vi "CMD git branch -v.vi"(8 "error in (no error)":errorcluster, 10 "git repo path":path=path "C:/Users/user/Desktop", 11 "git.exe path":path=path "C:/Program Files/Git/cmd/git.exe") -> (0 "error out":errorcluster, 2 "standard error":string, 3 "standard output":string, 5 "command operated":string)   [LabVIEW 2016]
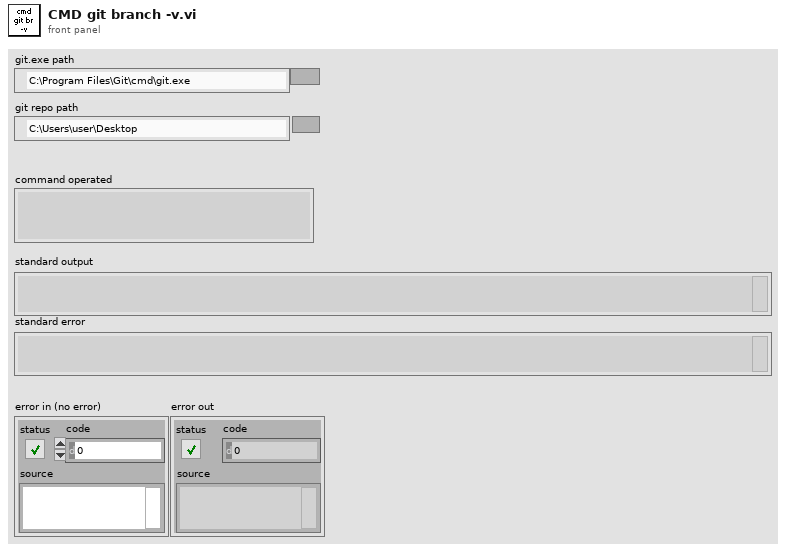
[diagram p1: front panel]
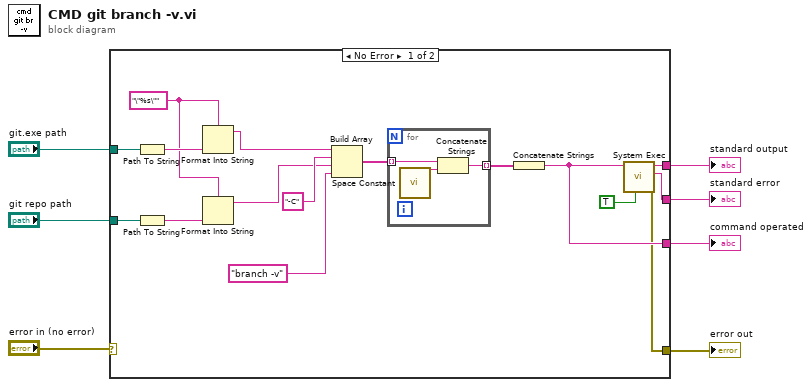
[diagram p0: block diagram]
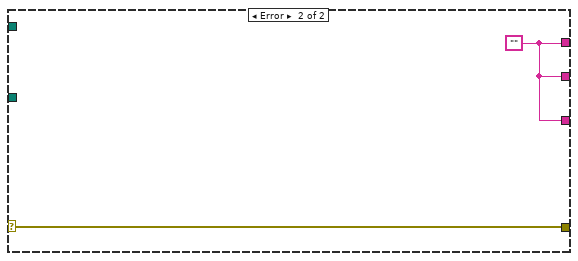
[diagram p2: hidden frame]
diagram:
  n1 = case shown="No Error" "error in (no error)" {
    selector: "error in (no error)" -> [_ w28]
    tunnel: "git repo path" -> [w19 _]
    tunnel: [w13 w27] -> w6
    tunnel: [w12 w27] -> w5
    tunnel: "git.exe path" -> [w10 _]
    tunnel: [w9 w27] -> w3
    tunnel: [w8 w28] -> w1
    frame No Error {
      w17 = "\"%s\"" ("format string")
      n2 = Path To String(path=w10) -> (string=w18:string)
      n3 = Path To String(path=w19) -> (string=w16:string)
      n4 = Format Into String(format string=w17, w18) -> (resulting string=w15:string)  [unwired: 2 in, 1 out]
      n5 = Format Into String(format string=w17, w16) -> (resulting string=w14:string)  [unwired: 2 in, 1 out]
      n6 = Build Array(w15, "-C" ("string"), w14, "branch -v" ("string")) -> (w21:string[])
      n7 = for {
        tunnel: w21 -> [w26] mode=indexing
        tunnel: [w24] -> w20 mode=indexing
        n8 = call <vilib>:"Space Constant.vi"() -> ("String"=w25:string)
        n9 = Concatenate Strings(w26, w25) -> (w24:string)
      }
      n10 = Concatenate Strings(w20) -> (w13:string)
      n11 = call <vilib>:"System Exec.vi"("run minimized? (F)"=TRUE, "command line"=w13) -> ("error out"=w8:errorcluster, "standard error"=w9:string, "standard output"=w12:string)  [unwired: 6 in, 1 out]
    }
    frame Error {
      w27 = ""
    }
  }
  "command operated" <- w6
  "standard output" <- w5
  "standard error" <- w3
  "error out" <- w1
